vi "Save Data.vi"(4 "file path (dialog if empty)":path, 6 "Save Data?":bool, 8 "error in (no error)":errorcluster, 9 "ERD Data":string[][](array[string])) -> (0 "error out":errorcluster)   [LabVIEW 2023]
uses:
  <vilib>/Utility/file.llb/Write Delimited Spreadsheet (string).vi
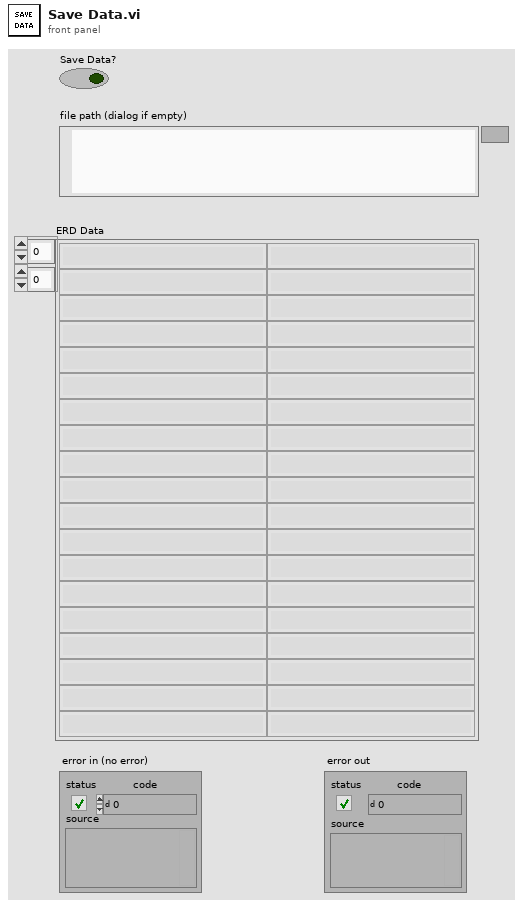
[diagram p1: front panel]
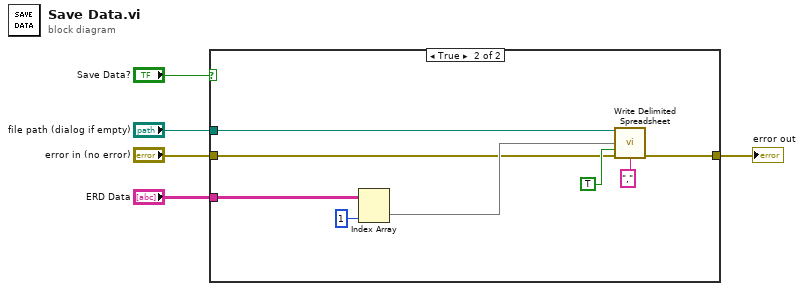
[diagram p0: block diagram]
diagram:
  n1 = case shown="True" "Save Data?" {
    tunnel: "ERD Data" -> [_ w13]
    tunnel: "error in (no error)" -> [w6 w9]
    tunnel: [w6 w8] -> w2
    tunnel: "file path (dialog if empty)" -> [_ w7]
    frame False {
    }
    frame True {
      n2 = Index Array(array=w13, index (col)=1 ("disabled index (col)")) -> (element=w11:string[])  [unwired: 1 in]
      n3 = call-poly <vilib>:"Write Delimited Spreadsheet.vi"("file path (dialog if empty)"=w7, "1D data"=w11, "append to file? (new file:F)"=TRUE, "error in (no error)"=w9, "delimiter (\\t)"="," ("delimiter (\\t)")) -> ("error out"=w8:errorcluster)  [unwired: 9 in, 1 out]
    }
  }
  "error out" <- w2
